vi "Message type.vi"(11 "IWelcomeHandler in":refnum<class "IWelcomeHandler.lvclass">) -> (2 "Internal message type":T1, 3 "IWelcomeHandler out":refnum<class "IWelcomeHandler.lvclass">)   [LabVIEW 2020, in "wamplv.lvlib" / "IWelcomeHandler.lvclass"]
uses:
  IWelcomeHandler.lvclass
  TypeDefs/Internal message type.ctl
  wamplv.lvlib
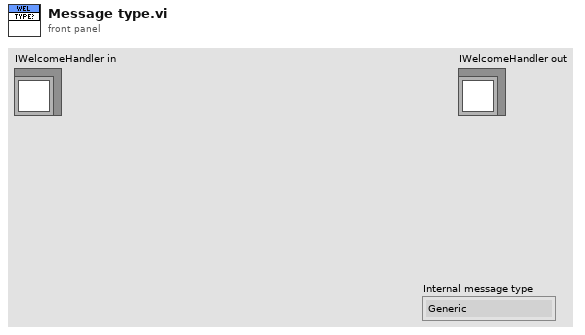
[diagram p1: front panel]
types:
  T1 = typedef "wamplv.lvlib/Internal message type.ctl" = enum16{"Generic", "Generic with write output", "Handle Result", "Handle Error", "Handle Abort", "Handle Welcome"}
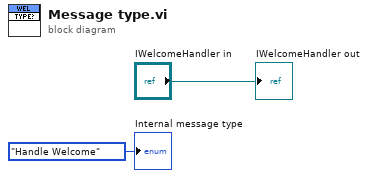
[diagram p0: block diagram]
diagram:
  "IWelcomeHandler out" <- "IWelcomeHandler in"
  "Internal message type" <- Internal_message_type."Handle Welcome" ("Internal message type")
